vi "add_twist_roslv.vi"(4 "Twist":T1, 5 "msg in":string) -> (2 "msg out":string)   [LabVIEW 2014]
doc: "Flattens a twist into a string"
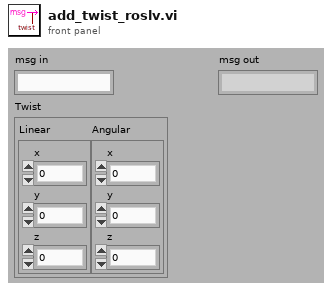
[diagram p1: front panel]
types:
  T1 = cluster{"Linear":cluster{"x":dbl, "y":dbl, "z":dbl}, "Angular":cluster{"x":dbl, "y":dbl, "z":dbl}}
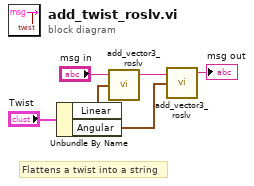
[diagram p0: block diagram]
diagram:
  # "Flattens a twist into a string"
  n1 = Unbundle By Name("Twist") -> ("Linear"=w4:cluster{"x":dbl, "y":dbl, "z":dbl}, "Angular"=w3:cluster{"x":dbl, "y":dbl, "z":dbl})
  n2 = call "add_vector3_roslv.vi"("Vector3"=w4, "msg in"="msg in") -> ("msg out"=w6:string)  [unwired: 3 in]
  n3 = call "add_vector3_roslv.vi"("Vector3"=w3, "msg in"=w6) -> ("msg out"=→"msg out":string)  [unwired: 3 in]
